vi "IV to tsv 3 columns.vi"(8 "experiment name":string, 9 "Iteration":i32, 10 "Sweep parameters":T1, 11 "output cluster":cluster{dbl[], dbl[], dbl[]}) -> ()   [LabVIEW 2016]
uses:
  <vilib>/MakerHub/Toolbox/LMH-Toolbox.lvlib
panel:
  out "concatenated string":string
  out "appended path":path
  out "appended array":dbl[][](array[numeric])
  out "spreadsheet string":string
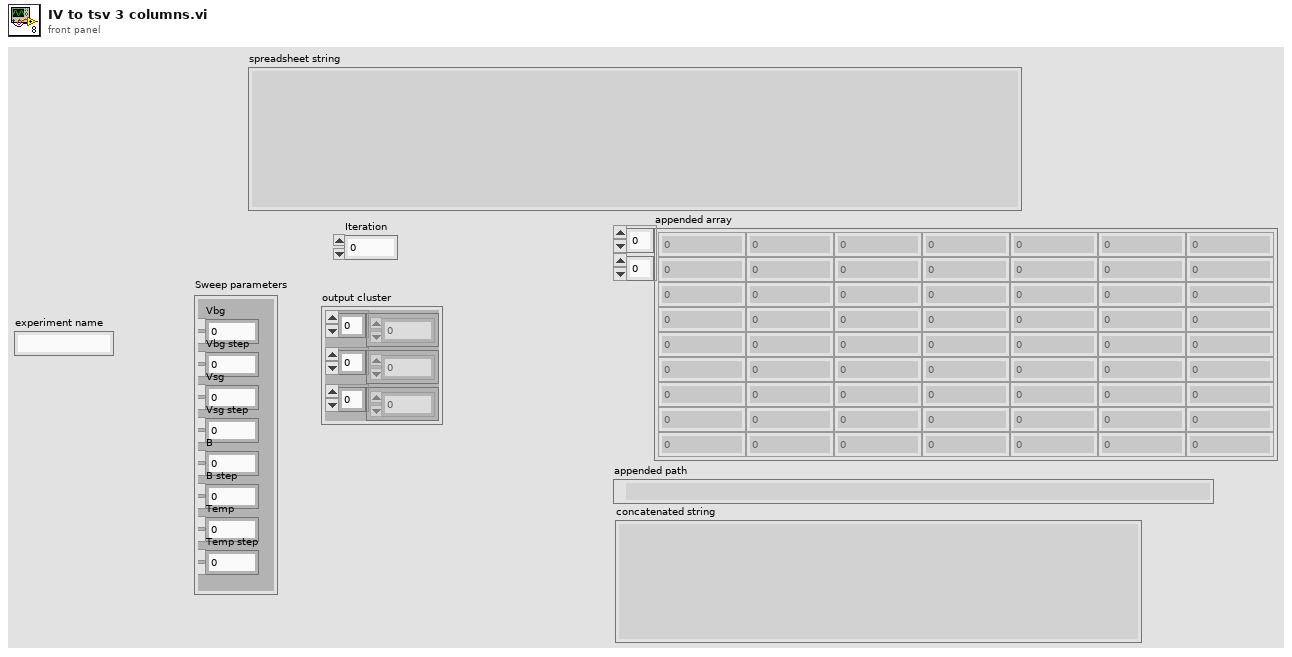
[diagram p1: front panel]
types:
  T1 = cluster{"Vbg":dbl, "Vbg step":dbl, "Vsg":dbl, "Vsg step":dbl, "B":dbl, "B step":dbl, "Temp":dbl, "Temp step":dbl}
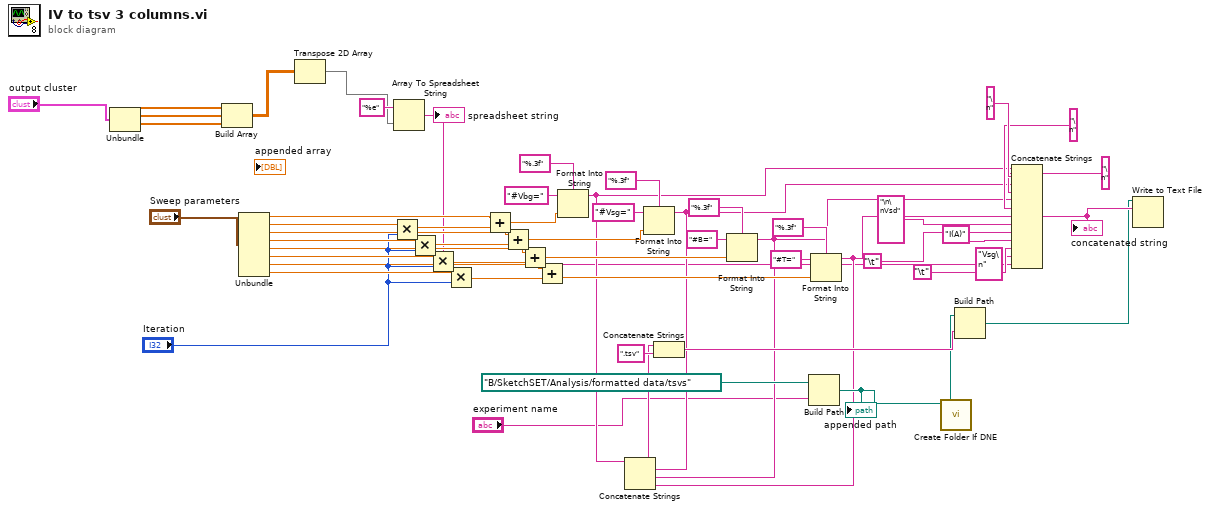
[diagram p0: block diagram]
diagram:
  n1 = Unbundle("output cluster") -> (w8:dbl[], w7:dbl[], w6:dbl[])
  n2 = Build Array(w8, w7, w6) -> (w2:dbl[][])
  n3 = Unbundle("Sweep parameters") -> ("Vbg"=w50:dbl, "Vbg step"=w54:dbl, "Vsg"=w48:dbl, "Vsg step"=w53:dbl, "B"=w46:dbl, "B step"=w52:dbl, "Temp"=w44:dbl, "Temp step"=w51:dbl)
  n4 = Transpose 2D Array(2D array=w2) -> (transposed array=w1:dbl[][])
  n5 = Multiply(x=w54, y="Iteration") -> (x*y=w49:dbl)
  n6 = Array To Spreadsheet String(array=w1, 3:"%e" ("format string")) -> (spreadsheet string=w3:string)  [unwired: 1 in]
  "spreadsheet string" <- w3
  n7 = Multiply(x=w53, y="Iteration") -> (x*y=w47:dbl)
  n8 = Multiply(x=w52, y="Iteration") -> (x*y=w45:dbl)
  n9 = Multiply(x=w51, y="Iteration") -> (x*y=w43:dbl)
  n10 = Add(x=w50, y=w49) -> (x+y=w41:dbl)
  n11 = Add(x=w48, y=w47) -> (x+y=w34:dbl)
  n12 = Add(x=w46, y=w45) -> (x+y=w33:dbl)
  n13 = Add(x=w44, y=w43) -> (x+y=w32:dbl)
  n14 = Format Into String(format string="%.3f", initial string="#Vbg=", w41) -> (resulting string=w17:string)  [unwired: 1 in, 1 out]
  n15 = Format Into String(format string="%.3f", initial string="#Vsg=", w34) -> (resulting string=w16:string)  [unwired: 1 in, 1 out]
  n16 = Format Into String(format string="%.3f", initial string="#B=", w33) -> (resulting string=w15:string)  [unwired: 1 in, 1 out]
  n17 = Build Path(base path=path "B:/SketchSET/Analysis/formatted data/tsvs", name or relative path="experiment name") -> (appended path=w22:path)
  "appended path" <- w22
  n18 = Format Into String(format string="%.3f", initial string="#T=", w32) -> (resulting string=w14:string)  [unwired: 1 in, 1 out]
  n19 = Concatenate Strings(w17, w16, w15, w14) -> (w13:string)
  n20 = Concatenate Strings(w13, ".tsv" ("string")) -> (w24:string)
  n21 = call <vilib>:"Create Folder If DNE.vi"("Folder Path"=w22) -> ("Dup Path"=w21:path)  [unwired: 9 in, 1 out]
  n22 = Build Path(base path=w21, name or relative path=w24) -> (appended path=w26:path)
  n23 = Concatenate Strings(w17, "\n" ("string"), w16, "\n" ("string"), w15, "\n" ("string"), w14, "\n\nVsd" ("string"), "\t", "I(A)" ("string"), "\t", "Vsg\n" ("string"), w3) -> (w28:string)
  "concatenated string" <- w28
  n24 = Write to Text File(file (use dialog)=w26, text=w28) -> ()  [unwired: 2 in, 3 out]
